vi "Robot Global Data.vi"() -> ()   [LabVIEW 2018]
doc: "This global VI can contain as many global variables as you need. Place a control on the panel, give it a good name. To read or write to it from a VI, drag the icon to the diagram of that VI. You can also drag from the project. Click on the node to change which global you access. You shouldn't have multiple locations writing to a global or it will cause a race-condition."
uses:
  <vilib>/Rock Robotics/WPI/Camera/WPI_CameraImageSize.ctl
  <vilib>/Rock Robotics/WPI/DriverStation/WPI_DriverStationRobotMode2.ctl
panel:
  in  "Collector Angle Down/Out":bool
  in  "Collector Angle Up/In":bool
  in  "HAB 3: Drive Module\n(FORWARD)":bool
  in  "HAB 3: All Cylinders":bool
  in  "HAB  3: Override Switches":bool
  in  "Hab 3: Front Cylinders":bool
  in  "HAB 3: Back Cylinders Only":bool
  in  "Collector Angle: Vertical":bool
  in  "Collector Angle: Dustpan Hover":bool
  in  "Kick Hatch (Hold)":bool
  in  "Hatch Retainer Up/Down":bool
  in  "Robot Mode":T1
  in  "image size":T2=enum."320x240"
  in  "Enable Vision":bool
  # "LEFT TRIGGER"
  # "RIGHT TRIGGER"
  # "Aux Controls :D"
  # "LEFT BUMPER"
  # "RIGHT BUMPER"
  # "Left Joystick"
  # "Right Joystick"
  # "Y-BUTTON"
  # "X-BUTTON"
  # "B-BUTTON"
  # "A-BUTTON"
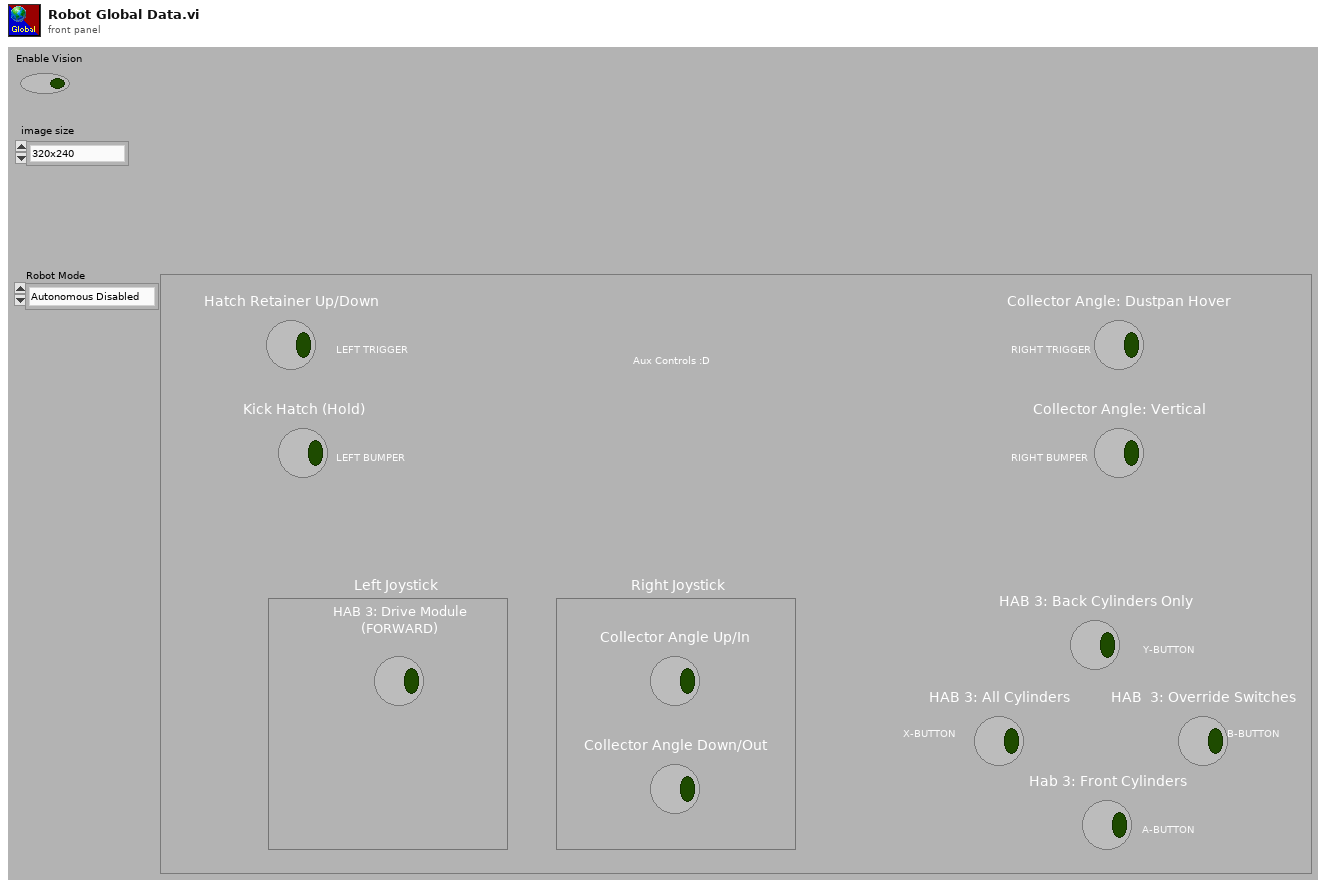
[diagram p1: front panel]
types:
  T1 = typedef "WPI_DriverStationRobotMode2.ctl" = enum16{"Autonomous Disabled", "Autonomous Enabled", "Teleop Disabled", "Teleop Enabled", "Disconnected", "Finish", "Test Disabled", "Test Enabled", "Emergency Stopped"}
  T2 = typedef "WPI_CameraImageSize.ctl" = enum16{"640x480", "320x240", "160x120", "Custom"}
diagram:
